vi "dg535 delay.vi"(0 "Delays (A,B,C,D)":dbl[](array[numeric]), 1 "VISA resource name":refnum<visa-resource-name>="GPIB0::15::INSTR", 3 "Modes":cluster{"A=":u32, "B=":u32, "C=":u32, "D=":u32} {"D=" scale=0.0..3.0; "C=" scale=0.0..3.0; "B=" scale=0.0..3.0; "A=" scale=0.0..3.0}, 4 "error in":errorcluster) -> (9 "error out":errorcluster)   [LabVIEW 2009]
doc: "This subVI sets the delay of the output channels relative to other channels or to the time reference T0 .\nControls A=, B= , C= and D= specify the reference channel and \nA, B, C, and D set the delay time in seconds .\nA Delay Linkage Error will be caused by an attempt to totally disconnect a time reference from T0 ."
panel:
  out "return count":u32
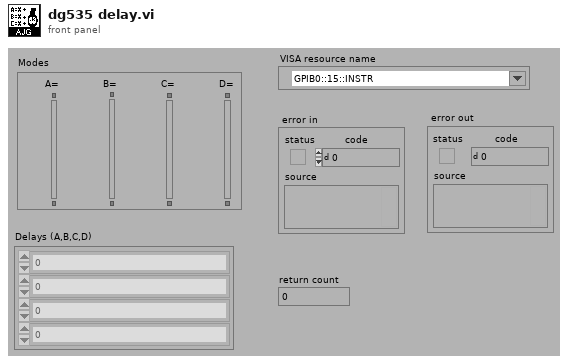
[diagram p1: front panel]
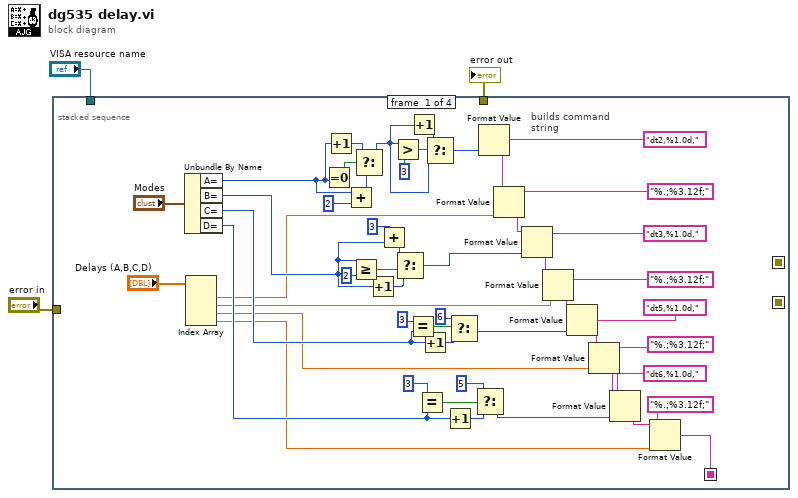
[diagram p0: block diagram]
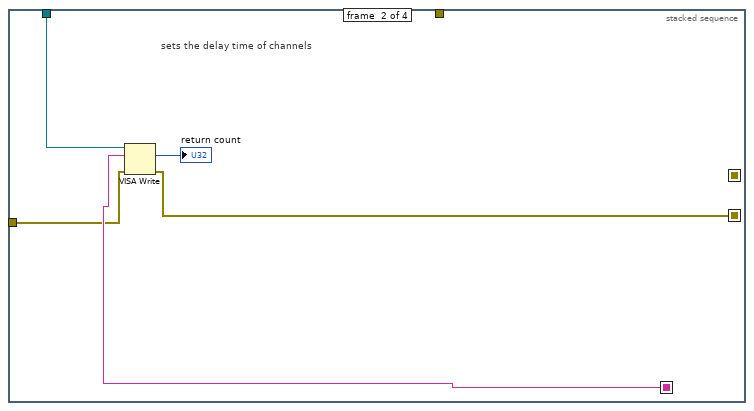
[diagram p2: hidden frame]
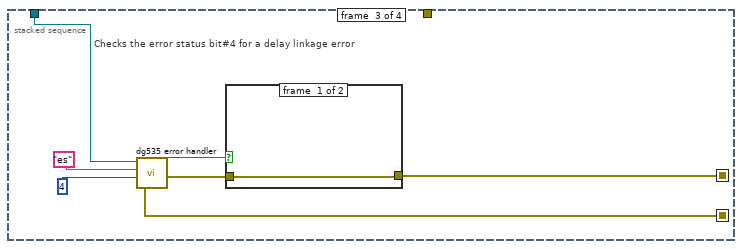
[diagram p3: hidden frame]
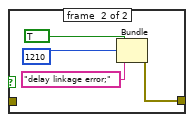
[diagram p4: hidden frame]
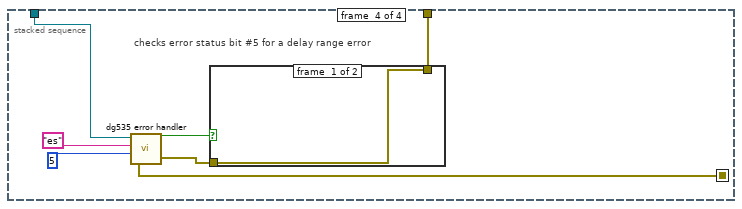
[diagram p5: hidden frame]
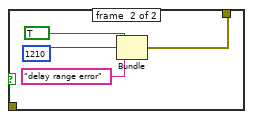
[diagram p6: hidden frame]
diagram:
  n1 = stacked-sequence {
    seq-local: [w40 _ _ _] -> [_ w58 _ _]
    seq-local: [_ w56 _ _] -> [_ _ w66 _]
    seq-local: [_ _ w63 _] -> [_ _ _ w73]
    tunnel: "error in" -> [_ w57 _ _]
    tunnel: [_ _ _ w76] -> w2
    tunnel: "VISA resource name" -> [_ w59 w60 w72]
    frame #0 {
      # "builds command\nstring"
      n2 = Unbundle By Name("Modes") -> ("A="=w12:u32, "B="=w11:u32, "C="=w10:u32, "D="=w9:u32)
      n3 = Index Array(array="Delays (A,B,C,D)") -> (element #1=w7:dbl, element #2=w6:dbl, element #3=w5:dbl, element #4=w4:dbl)  [unwired: 4 in]
      n4 = Equal To 0?(x=w12) -> (x = 0?=w23:bool)
      n5 = Increment(x=w12) -> (x+1=w15:u32)
      n6 = Add(x=w12, y=2) -> (x+y=w21:u32)
      n7 = Greater Or Equal?(x=w11, y=2) -> (x >= y?=w26:bool)
      n8 = Select(t=w15, s=w23, f=w21) -> (s? t:f=w14:u32)
      n9 = Increment(x=w11) -> (x+1=w24:u32)
      n10 = Add(x=3, y=w11) -> (x+y=w27:u32)
      n11 = Greater?(x=w14, y=3) -> (0:w19:bool)
      n12 = Select(t=w27, s=w26, f=w24) -> (s? t:f=w25:u32)
      n13 = Equal?(x=3, y=w10) -> (x = y?=w33:bool)
      n14 = Increment(x=w14) -> (x+1=w18:u32)
      n15 = Equal?(x=3, y=w9) -> (x = y?=w37:bool)
      n16 = Increment(x=w10) -> (x+1=w30:u32)
      n17 = Select(t=w18, s=w19, f=w14) -> (s? t:f=w17:u32)
      n18 = Increment(x=w9) -> (x+1=w31:u32)
      n19 = Select(t=6, s=w33, f=w30) -> (s? t:f=w29:u32)
      n20 = Select(t=5, s=w37, f=w31) -> (s? t:f=w35:u32)
      n21 = Format Value(format string="dt2,%1.0d,", value (0)=w17) -> (output string=w49:string)  [unwired: 1 out]
      n22 = Format Value(string ("")=w49, format string="%.;%3.12f;", value (0)=w7) -> (output string=w48:string)
      n23 = Format Value(string ("")=w48, format string="dt3,%1.0d,", value (0)=w25) -> (output string=w51:string)
      n24 = Format Value(string ("")=w51, format string="%.;%3.12f;", value (0)=w6) -> (output string=w39:string)
      n25 = Format Value(string ("")=w39, format string="dt5,%1.0d,", value (0)=w29) -> (output string=w43:string)
      n26 = Format Value(string ("")=w43, format string="%.;%3.12f;", value (0)=w5) -> (output string=w41:string)
      n27 = Format Value(string ("")=w41, format string="dt6,%1.0d,", value (0)=w35) -> (output string=w46:string)
      n28 = Format Value(string ("")=w46, format string="%.;%3.12f;", value (0)=w4) -> (output string=w40:string)
    }
    frame #1 {
      # "sets the delay time of channels"
      n29 = VISA Write(VISA resource name=w59, write buffer=w58, error in (no error)=w57) -> (return count=→"return count":u32, error out=w56:errorcluster)  [unwired: 1 out]
    }
    frame #2 {
      # "Checks the error status bit#4 for a delay linkage error"
      n30 = call "dg535 error handler.vi"("error in"=w66, "check bit #"=4, "command string"="es", "VISA resource name"=w60) -> ("error out"=w64:errorcluster, "error found"=w65:bool)
      n31 = case shown="True" w65 {
        tunnel: w64 -> [w67 _]
        tunnel: [w67 w68] -> w63
        frame #0 {
        }
        frame #1 {
          n32 = Bundle(TRUE, 1210, "delay linkage error;") -> (w68:errorcluster)  [unwired: 1 out]
        }
      }
    }
    frame #3 {
      # "checks error status bit #5 for a delay range error"
      n33 = call "dg535 error handler.vi"("error in"=w73, "check bit #"=5, "command string"="es", "VISA resource name"=w72) -> ("error out"=w77:errorcluster, "error found"=w78:bool)
      n34 = case shown="True" w78 {
        tunnel: w77 -> [w79 _]
        tunnel: [w79 w80] -> w76
        frame #0 {
        }
        frame #1 {
          n35 = Bundle(TRUE, 1210, "delay range error") -> (w80:errorcluster)  [unwired: 1 out]
        }
      }
    }
  }
  "error out" <- w2
